vi "Human Interface.vi"   [LabVIEW 2013]
uses:
  Systems/Drive/Drive Global.vi
  Systems/Cannon/Cannon Global.vi
  Systems/Orientation/Oritentation Global.vi
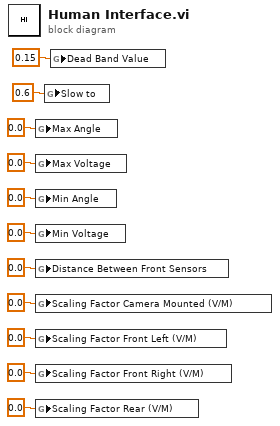
[diagram p0: block diagram]
diagram:
  n1 = global write "Cannon Global.vi" "Max Angle"(0.0) -> ()
  n2 = global write "Cannon Global.vi" "Max Voltage"(0.0) -> ()
  n3 = global write "Cannon Global.vi" "Min Angle"(0.0) -> ()
  n4 = global write "Cannon Global.vi" "Min Voltage"(0.0) -> ()
  n5 = global write "Oritentation Global.vi" "Distance Between Front Sensors"(0.0 ("Distance Between Front Sensors")) -> ()
  n6 = global write "Oritentation Global.vi" "Scaling Factor Camera Mounted (V/M)"(0.0 ("Distance Between Front Sensors")) -> ()
  n7 = global write "Oritentation Global.vi" "Scaling Factor Front Left (V/M)"(0.0 ("Distance Between Front Sensors")) -> ()
  n8 = global write "Oritentation Global.vi" "Scaling Factor Front Right (V/M)"(0.0 ("Distance Between Front Sensors")) -> ()
  n9 = global write "Oritentation Global.vi" "Scaling Factor Rear (V/M)"(0.0 ("Distance Between Front Sensors")) -> ()
  n10 = global write "Drive Global.vi" "Slow to"(0.6) -> ()
  n11 = global write "Drive Global.vi" "Dead Band Value"(0.15 ("Dead Band Value")) -> ()
